vi "Unique Number Array Builder.vi"() -> ()   [LabVIEW 2025]
panel:
  out "Minimum value":dbl
  out "Maximum value":dbl
  out "Sorted array":dbl[](array[numeric])
  out "Array":dbl[](array[numeric])
  in  "Number to input":dbl
  in  "stop":bool
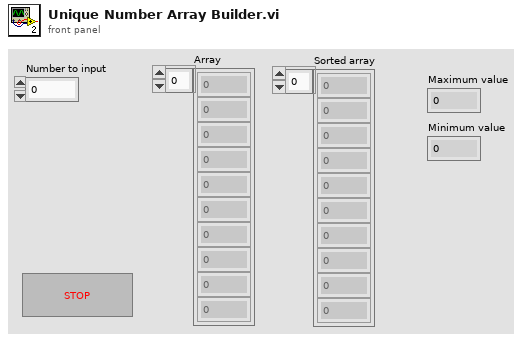
[diagram p1: front panel]
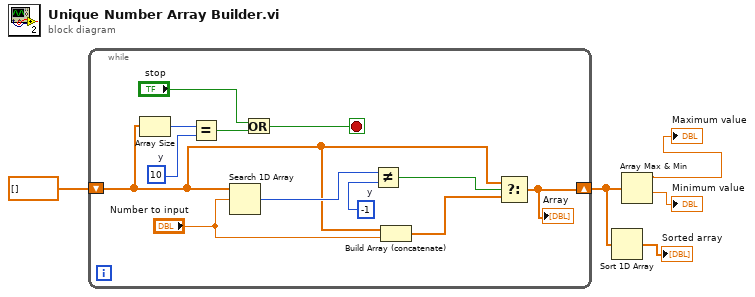
[diagram p0: block diagram]
diagram:
  n1 = while {
    shift-right: [w17] -> w4
    shift-left: dbl[] [] -> [w6]
    stop <- w7 stop-if-true
    w10 = 10  # y
    w14 = -1  # y
    n2 = Array Size(array=w6) -> (size(s)=w11:i32)
    n3 = Equal?(x=w11, y=w10) -> (x = y?=w9:bool)
    n4 = Search 1D Array(1D array=w6, element="Number to input") -> (index of element=w13:i32)  [unwired: 1 in]
    n5 = Or(x="stop", y=w9) -> (x .or. y?=w7:bool)
    n6 = Not Equal?(x=w13, y=w14) -> (x != y?=w12:bool)
    n7 = Build Array (concatenate) "Build Array"(w6, "Number to input") -> (w16:dbl[])
    n8 = Select(t=w6, s=w12, f=w16) -> (s? t:f=w17:dbl[])
    "Array" <- w17
  }
  n9 = Sort 1D Array(array=w4) -> (sorted array=→"Sorted array":dbl[])
  n10 = Array Max & Min(array=w4) -> (max value=→"Maximum value":dbl, min value=→"Minimum value":dbl)  [unwired: 2 out]
